vi "setUp.vi"(8 "error in (no error)":errorcluster, 11 "reference in":refnum<class "RSI Module Unit Tests.lvclass">) -> (0 "error out":errorcluster, 3 "reference out":refnum<class "RSI Module Unit Tests.lvclass">)   [LabVIEW 2017, in "RSI Module Unit Tests.lvclass"]
doc: "setUp runs prior to the test method during test execution. Use this method to initialize any object data required by your tests."
uses:
  RSI Module Unit Tests.lvclass
  C:/Program Files (x86)/National Instruments/LabVIEW 2017/vi.lib/addons/_JKI Toolkits/VI Tester/TestCase.llb/TestCase.lvclass
  <vilib>/addons/_JKI Toolkits/VI Tester/TestCase.llb/TestCase.lvclass
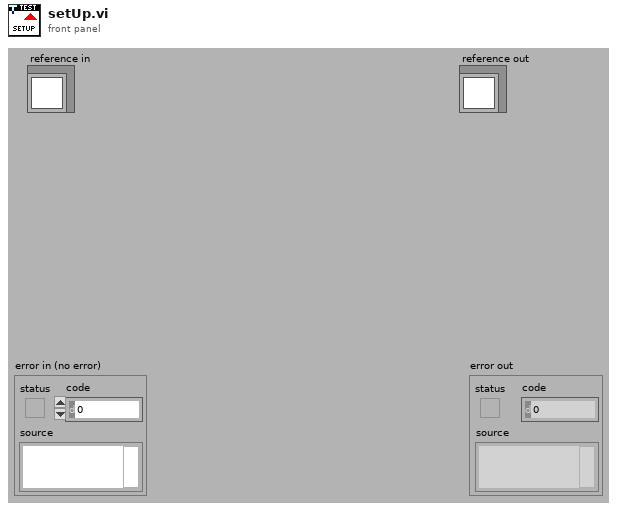
[diagram p1: front panel]
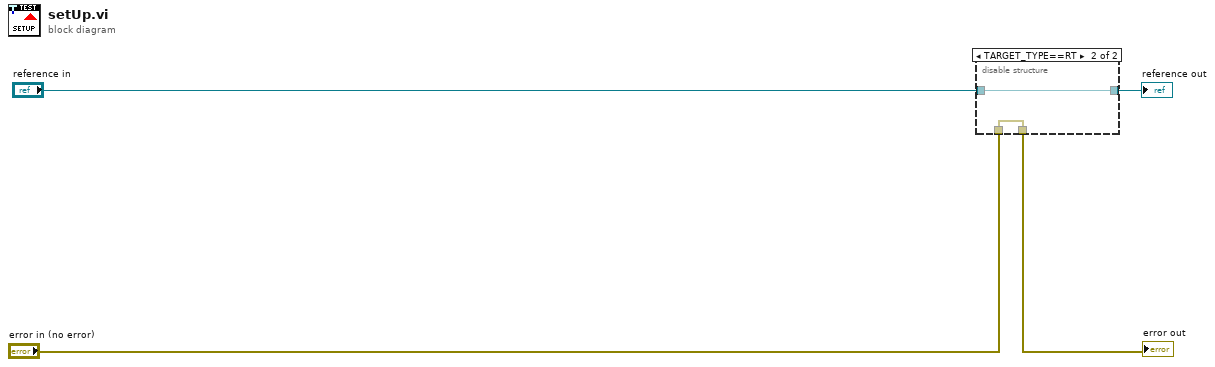
[diagram p0: block diagram]
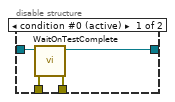
[diagram p2: hidden frame]
diagram:
  n1 = disable-structure shown="TARGET_TYPE==RT" {
    disable-tunnel: "error in (no error)" -> [w8 w9]
    disable-tunnel: [w7 w9] -> w3
    disable-tunnel: [w6 w10] -> w2
    disable-tunnel: "reference in" -> [w5 w10]
    frame condition #0 (active) {
      n2 = call <vilib>:"WaitOnTestComplete.vi"("error in (no error)"=w8, "TestCase in"=w5) -> ("error out"=w7:errorcluster, "TestCase out"=w6:refnum<class "RSI Module Unit Tests.lvclass">)  [unwired: 8 in]
    }
    frame condition #1 {
    }
  }
  "error out" <- w3
  "reference out" <- w2
